vi "Arcsec to Rad.vi"(1 "Arcsec":dbl) -> (0 "rad":dbl)   [LabVIEW 2018]
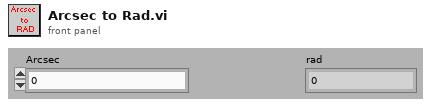
[diagram p1: front panel]
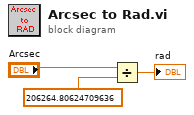
[diagram p0: block diagram]
diagram:
  n1 = Divide(x="Arcsec", y=206264.80624709636) -> (x/y=→"rad":dbl)
